vi "axex_get_list_of_workbooks_proc.vi"(8 "error in":errorcluster, 11 "names ring ref":refnum<vi>) -> (0 "error out":errorcluster, 1 "Excel not running":bool, 2 "names":string[](array[string]), 3 "full paths":string[](array[string]))   [LabVIEW 2020, in "AX Excel.lvlib"]
doc: "Returns list of opened workbooks. Will not generate error."
uses:
  AX Excel.lvlib
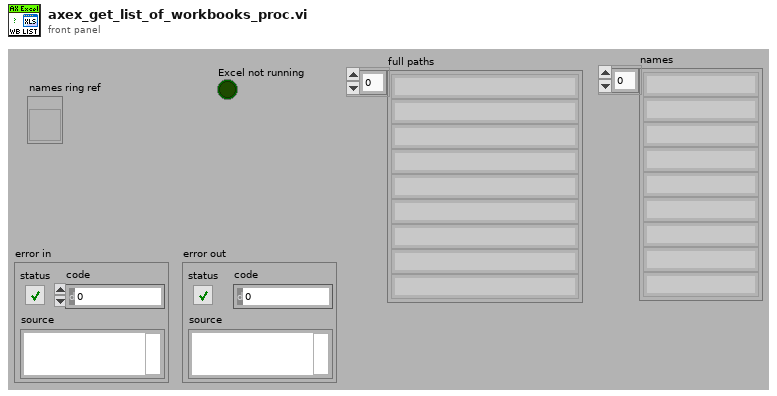
[diagram p1: front panel]
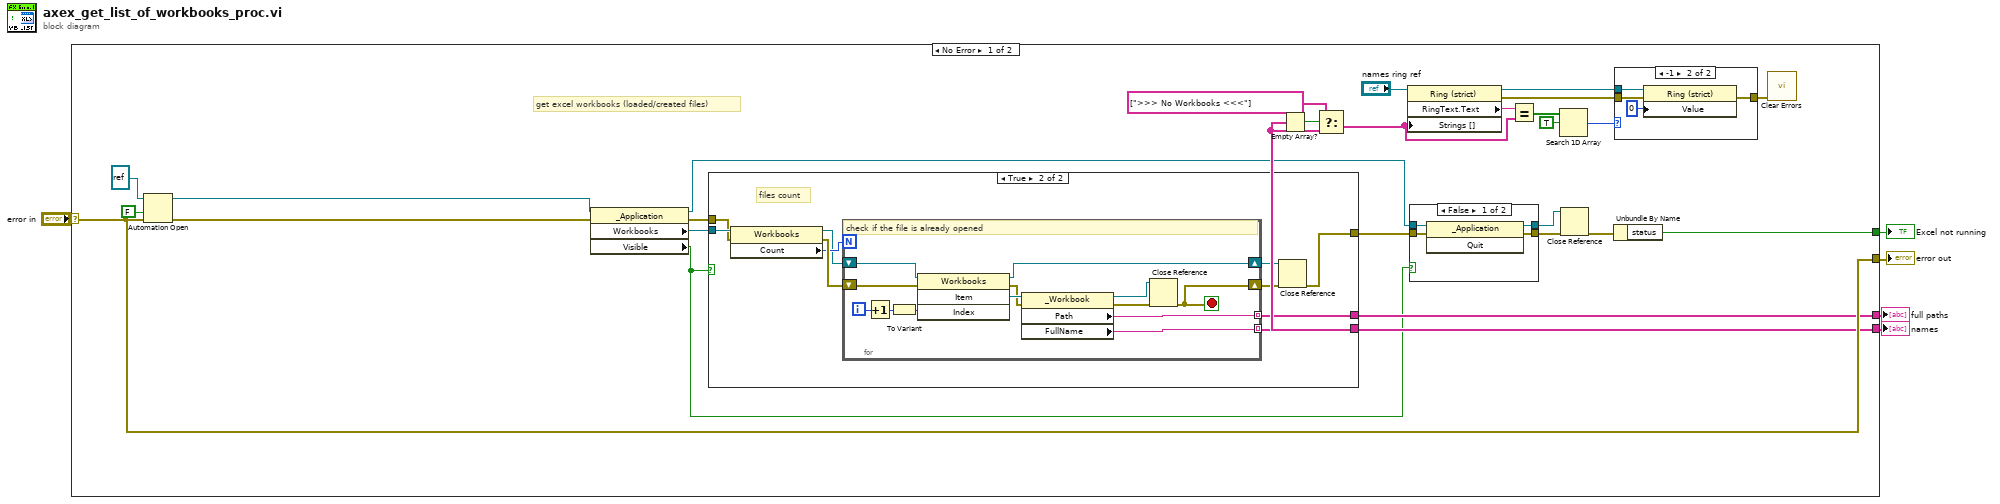
[diagram p0: block diagram]
diagram:
  n1 = case shown="No Error" "error in" {
    selector: "error in" -> [w29 w68]
    tunnel: [w29 w68] -> w5
    tunnel: [w28 _] -> w3
    tunnel: [w27 _] -> w2
    tunnel: [w25 _] -> w1
    frame No Error {
      # "get excel workbooks (loaded/created files)"
      n2 = Automation Open(error in (no error)=w29, Automation Refnum=refnum<k7> refnum ("Excel._Application"), 9:FALSE ("open new instance (false)")) -> (Automation Refnum=w7:refnum<k7>, error out=w8:errorcluster)  [unwired: 1 in]
      n3 = property class="_Application"(reference=w7, error in=w8) -> (reference out=w9:refnum<k7>, error out=w30:errorcluster, "Workbooks"=w31:refnum<k7>, "Visible"=w10:bool)
      n4 = case shown="True" w10 {
        tunnel: w31 -> [_ w41]
        tunnel: w30 -> [w33 w40]
        tunnel: [_ w36] -> w27
        tunnel: [_ w35] -> w25
        tunnel: [w33 w34] -> w12
        frame False {
        }
        frame True {
          # "files count"
          n5 = property class="Workbooks"(reference=w41, error in=w40) -> (reference out=w39:refnum<k7>, error out=w43:errorcluster, "Count"=w42:i32)
          n6 = for {
            N: w42 -> [_]
            shift-right: [w46] -> w38
            shift-left: w43 -> [w55]
            shift-right: [w47] -> w37
            shift-left: w39 -> [w53]
            tunnel: [w45] -> w36 mode=indexing
            tunnel: [w44] -> w35 mode=indexing
            i -> [w51]
            stop <- w46 stop-if-true
            # "check if the file is already opened"
            n7 = Increment(x=w51) -> (x+1=w50:i32)
            n8 = To Variant(anything=w50) -> (Variant=w52:variant)
            n9 = invoke class="Workbooks" method="Item"(reference=w53, error in=w55, "Index"=w52) -> (reference out=w47:refnum<k7>, error out=w54:errorcluster, "Item"=w56:refnum<k7>)  [unwired: 1 in, 1 out]
            n10 = property class="_Workbook"(reference=w56, error in=w54) -> (reference out=w48:refnum<k7>, error out=w49:errorcluster, "Path"=w45:string, "FullName"=w44:string)
            n11 = Close Reference(reference=w48, error in (no error)=w49) -> (error out=w46:errorcluster)
          }
          n12 = Close Reference(reference=w37, error in (no error)=w38) -> (error out=w34:errorcluster)
        }
      }
      n13 = Empty Array?(array=w25) -> (empty?=w24:bool)
      n14 = Select(t=string[] [">>> No Workbooks <<<"], s=w24, f=w25) -> (s? t:f=w21:string[])
      n15 = property class="Ring (strict)"(reference="names ring ref", "Strings []"=w21) -> (reference out=w17:refnum<vi>, error out=w16:errorcluster, "RingText.Text"=w22:string)  [unwired: 1 in]
      n16 = case shown="False" w10 {
        tunnel: [w60 w62] -> w13
        tunnel: w12 -> [w59 w62]
        tunnel: w9 -> [w58 w61]
        tunnel: [w57 w61] -> w11
        frame False {
          n17 = invoke class="_Application" method="Quit"(reference=w58, error in=w59) -> (reference out=w57:refnum<k7>, error out=w60:errorcluster)  [unwired: 1 in, 1 out]
        }
        frame True {
        }
      }
      n18 = Equal?(x=w22, y=w21) -> (x = y?=w20:bool[])
      n19 = Search 1D Array(1D array=w20, element=TRUE) -> (index of element=w18:i32)  [unwired: 1 in]
      n20 = Close Reference(reference=w11, error in (no error)=w13) -> (error out=w6:errorcluster)
      n21 = Unbundle By Name(w6) -> ("status"=w28:bool)
      n22 = case shown="-1" w18 {
        tunnel: w17 -> [_ w67]
        tunnel: w16 -> [w63 w66]
        tunnel: [w63 w65] -> w15
        frame Default {
        }
        frame -1 {
          n23 = property class="Ring (strict)"(reference=w67, error in=w66, "Value"=u16 0) -> (error out=w65:errorcluster)  [unwired: 1 out]
        }
      }
      n24 = call <vilib>:"Clear Errors.vi"("error in (no error)"=w15) -> ()  [unwired: 5 in, 2 out]
    }
    frame Error {
    }
  }
  "error out" <- w5
  "Excel not running" <- w3
  "full paths" <- w2
  "names" <- w1
